vi "Teleop.vi"() -> (1 "Stop program and write to file":bool, 2 "SWITCH TO AUTONOMOUS 2":bool, 3 "output cluster":T1)   [LabVIEW 2014]
panel:
  in  "Defense?":string(combo)="None"
  in  "Can they catch?":string(combo)="No"
  in  "SWITCH TO AUTONOMOUS":bool
  in  "Stop Program and Write to File":bool
  in  "Can they pick up the ball?":string(combo)="No"
  in  "Missed Shots":dbl
  in  "Comments":string
  in  "Over Truss With Catch":dbl
  in  "Helps":dbl
  in  "Under the Truss Pass":dbl
  in  "Over the Truss Pass":dbl
  in  "Bottom Goal":dbl
  in  "Top Goal":dbl
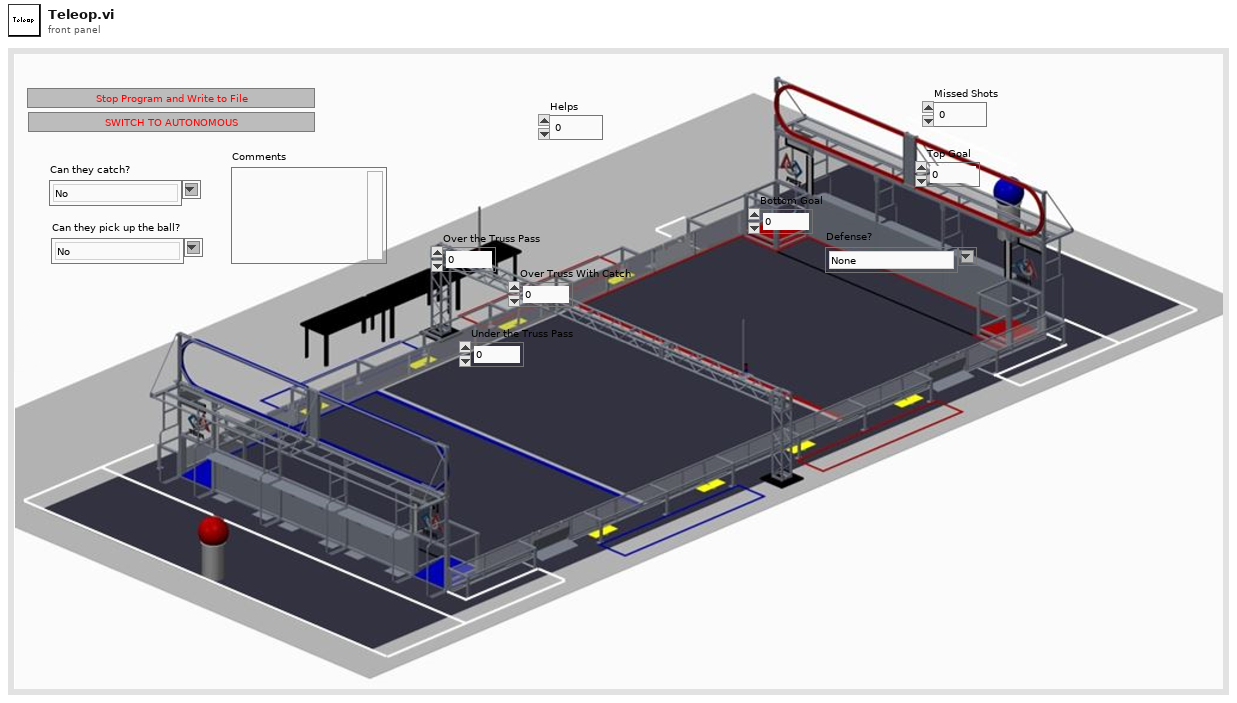
[diagram p1: front panel]
types:
  T1 = cluster{"Top Goal":dbl, "Bottom Goal":dbl, "Missed Shots":dbl, "Total":dbl, "Helps":dbl, "Over Truss With Catch":dbl, "Over the Truss Pass":dbl, "Under the Truss Pass":dbl, "Can they pick up the ball?":string, "Can they catch?":string, "Defense?":string, "Comments":string}
  T2 = cluster{dbl, "Bottom Goal":dbl, "Missed Shots":dbl, dbl, dbl, dbl, dbl, "Under the Truss Pass":dbl, "Can they pick up the ball?":string, "Can they catch?":string, "Defense?":string, "Comments":string}
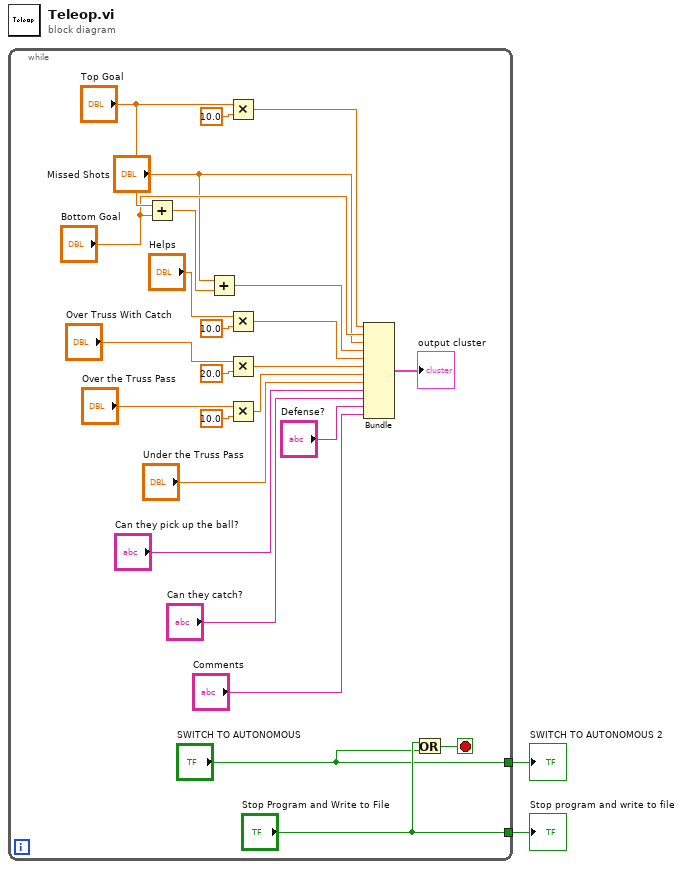
[diagram p0: block diagram]
diagram:
  n1 = while {
    tunnel: ["SWITCH TO AUTONOMOUS"] -> w2
    tunnel: ["Stop Program and Write to File"] -> w1
    stop <- w4 stop-if-true
    n2 = Add(x="Top Goal", y="Bottom Goal") -> (x+y=w24:dbl)
    n3 = Add(x="Missed Shots", y=w24) -> (x+y=w23:dbl)
    n4 = Multiply(x="Top Goal", y=10.0) -> (x*y=w25:dbl)
    n5 = Multiply(x="Helps", y=10.0) -> (x*y=w17:dbl)
    n6 = Multiply(x="Over Truss With Catch", y=20.0) -> (x*y=w14:dbl)
    n7 = Multiply(x="Over the Truss Pass", y=10.0) -> (x*y=w11:dbl)
    n8 = Bundle(w25, "Bottom Goal"="Bottom Goal", "Missed Shots"="Missed Shots", w23, w17, w14, w11, "Under the Truss Pass"="Under the Truss Pass", "Can they pick up the ball?"="Can they pick up the ball?", "Can they catch?"="Can they catch?", "Defense?"="Defense?", "Comments"="Comments") -> (→"output cluster":T2)  [unwired: 1 in]
    n9 = Or(x="Stop Program and Write to File", y="SWITCH TO AUTONOMOUS") -> (x .or. y?=w4:bool)
  }
  "Stop program and write to file" <- w1
  "SWITCH TO AUTONOMOUS 2" <- w2
